vi "PDC_GetColorTempBase.vi"(8 "error in (no error)":errorcluster, 10 "ChildNo":u32, 11 "DeviceNo":u32) -> (0 "error out":errorcluster, 1 "Max":u32, 2 "Base":u32, 3 "ReturnValue":u32, 4 "ErrorCode":u32)   [LabVIEW 2015]
doc: "This VI retrieves the reference value that can be used by the color temperature status setting of the specified child device."
uses:
  PDCLIB.dll
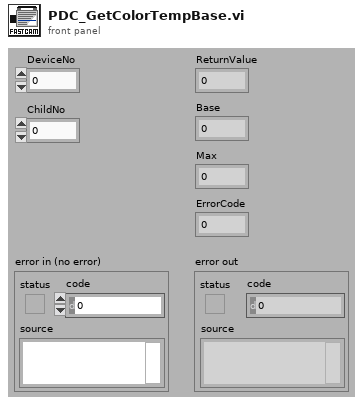
[diagram p1: front panel]
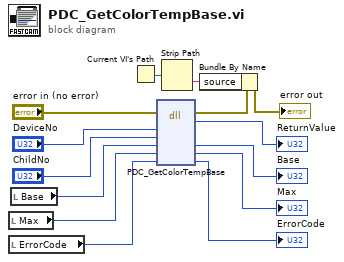
[diagram p0: block diagram]
diagram:
  n1 = local read "Max"() -> (w6:u32)
  n2 = local read "ErrorCode"() -> (w11:u32)
  n3 = local read "Base"() -> (w7:u32)
  n4 = Current VI's Path() -> (path=w3:path)
  n5 = dll-call lib="PDCLIB.dll" fn="PDC_GetColorTempBase"(error in="error in (no error)", "nDeviceNo"="DeviceNo", "nChildNo"="ChildNo", "pBase"=w7, "pMax"=w6, "pErrorCode"=w11) -> (error out=w2:errorcluster, "return type"=→"ReturnValue":u32, "pBase"=→"Base":u32, "pMax"=→"Max":u32, "pErrorCode"=→"ErrorCode":u32)  [unwired: 4 in, 1 out]
  n6 = Strip Path(path=w3) -> (name=w4:string)  [unwired: 1 out]
  n7 = Bundle By Name(cluster=w2, "source"=w4) -> (→"error out":errorcluster)
